vi "Timelapse viewer buttons disabled state.vi"(8 "error in (no error)":errorcluster, 10 "Disabled":T1(ring)) -> (0 "error out":errorcluster)   [LabVIEW 2013]
uses:
  Globals/gl_Time series viewer globals.vi
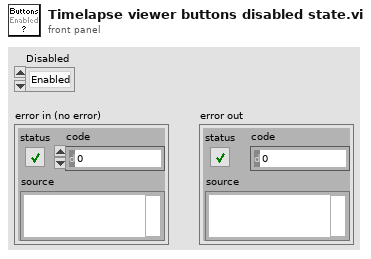
[diagram p1: front panel]
types:
  T1 = enum8{"Enabled", "Disabled", "Disabled and Grayed Out"}
  T2 = typedef "Timelapse viewer refs.ctl" = cluster{"This VI":refnum<vi>, "AVI Mode ind":refnum<vi>, "Play":refnum<vi>, "Stop":refnum<vi>, "Back":refnum<vi>, "Scrollbar":refnum<vi>, "Video length info":refnum<vi>, "Expected speed values":refnum<vi>, "Intensity":refnum<vi>, "Path":refnum<vi>, "Selection sliders":refnum<vi>, "Speed Graph ref":refnum<vi>, "Frame rate set (fps)":refnum<vi>}
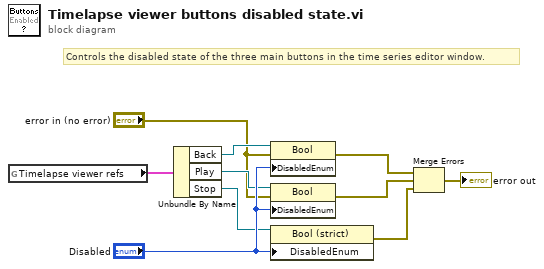
[diagram p0: block diagram]
diagram:
  # "Controls the disabled state of the three main buttons in the time series editor window."
  n1 = global read "gl_Time series viewer globals.vi" "Timelapse viewer refs"() -> (w1:T2)
  n2 = Unbundle By Name(w1) -> ("Back"=w5:refnum<vi>, "Play"=w6:refnum<vi>, "Stop"=w7:refnum<vi>)
  n3 = property on="Property Node" class="Bool"(reference=w5, error in="error in (no error)", "DisabledEnum"="Disabled") -> (error out=w3:errorcluster)  [unwired: 1 out]
  n4 = property on="Property Node" class="Bool"(reference=w6, error in="error in (no error)", "DisabledEnum"="Disabled") -> (error out=w4:errorcluster)  [unwired: 1 out]
  n5 = property on="Property Node" class="Bool (strict)"(reference=w7, "DisabledEnum"="Disabled") -> (error out=w9:errorcluster)  [unwired: 1 in, 1 out]
  n6 = Merge Errors(w3, w4, w9) -> (→"error out":errorcluster)
